vi "HAL camera initialize.vi"() -> (0 "error out":errorcluster)   [LabVIEW 2011]
uses:
  Cascade-specific globals.vi
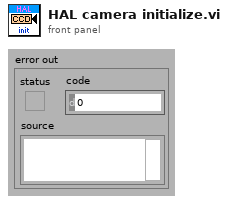
[diagram p1: front panel]
types:
  T1 = cluster{"Camera Handle":u32, "Pulser Handle":u32, "File Handle":u32, "Display Handle":u32, "Image Handle":u32}
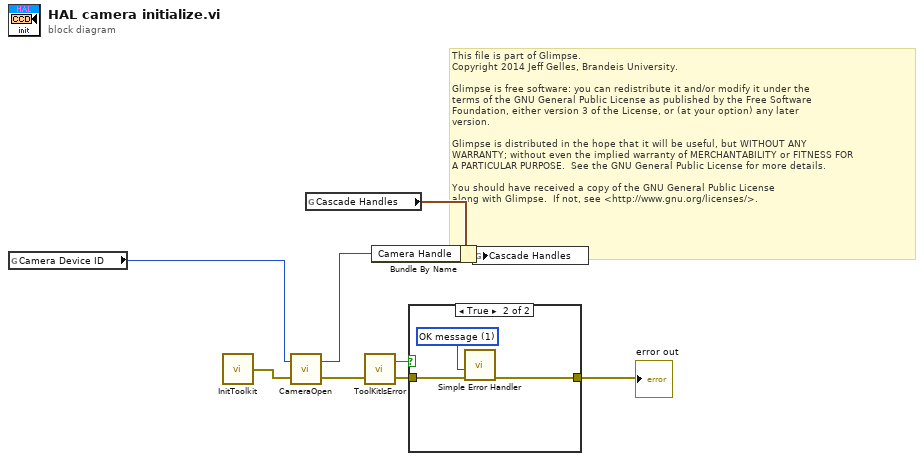
[diagram p0: block diagram]
diagram:
  # "This file is part of Glimpse. \nCopyright 2014 Jeff Gelles, Brandeis University.    \n\nGlimpse is free software: you can redistribute it and/or modify it under the \nterms of the GNU General Public License as published by the Free Software \nFoundation, either version 3 of the License, or (at your option) any later \nversion.\n\nGlimpse is distributed in the hope that it will be useful, but WITHOUT ANY \nWARRANTY; without even the implied warranty of MERCHANTABILITY or FITNESS FOR \nA PARTICULAR PURPOSE.  See the GNU General Public License for more details.\n\nYou should have received a copy of the GNU General Public License\nalong with Glimpse.  If not, see <http://www.gnu.org/licenses/>."
  n1 = global read "Cascade-specific globals.vi" "Camera Device ID"() -> (w4:u32)
  n2 = call <userlib>:"InitToolkit.vi"() -> ("error out"=w9:errorcluster)  [unwired: 1 in]
  n3 = call <userlib>:"CameraOpen.vi"("error in"=w9, "Camera Device ID"=w4) -> ("error out"=w8:errorcluster, "Camera Handle"=w1:u32)
  n4 = global read "Cascade-specific globals.vi" "Cascade Handles"() -> (w3:T1)
  n5 = call <userlib>:"ToolKitIsError.vi"("error in"=w8) -> ("error out"=w6:errorcluster, "Error Flag"=w7:bool)  [unwired: 1 in]
  n6 = Bundle By Name(cluster=w3, "Camera Handle"=w1) -> (w2:T1)
  n7 = case shown="True" w7 {
    tunnel: w6 -> [w10 w13]
    tunnel: [w10 w12] -> w5
    frame False {
    }
    frame True {
      w11 = u16 1 items=["no dialog", "OK message", "continue or stop message"] ("type of dialog (OK msg:1)")
      n8 = call <vilib>:"Simple Error Handler.vi"("type of dialog (OK msg:1)"=w11, "error in (no error)"=w13) -> ("error out"=w12:errorcluster)  [unwired: 7 out]
    }
  }
  "error out" <- w5
  n9 = global write "Cascade-specific globals.vi" "Cascade Handles"(w2) -> ()
